vi "Set Result Collector.vi"(8 "error in (no error)":errorcluster, 10 "Report Generator":refnum<class "Result Collector.lvclass">, 11 "Icon Decorator In":refnum<class "Icon Decorator.lvclass">) -> (0 "error out":errorcluster, 3 "Icon Decorator Out":refnum<class "Icon Decorator.lvclass">)   [LabVIEW 2020, in "Icon Decorator.lvclass"]
uses:
  Icon Decorator.lvclass
  C:/Users/anton/Documents/GitHub/LUnit/source/Application Framework/Process Classes/Process/Process.lvclass
  Result Collector/Result Collector.lvclass
  Application Framework/Process Classes/Process/Process.lvclass/Process.ctl
  Application Framework/Process Classes/Process/Process.lvclass
  Result Classes/Method Result/Method Result.lvclass
  Result Classes/Test Case Result/Test Case Result.lvclass
  Result Classes/Test Suite Result/Test Suite Result.lvclass
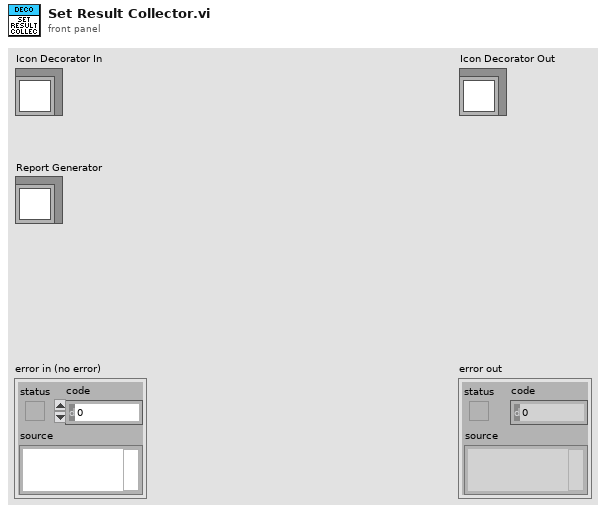
[diagram p1: front panel]
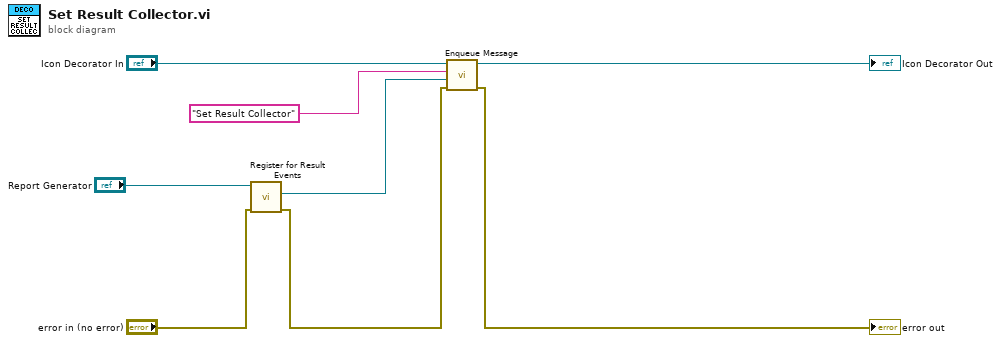
[diagram p0: block diagram]
diagram:
  n1 = call "Register for Result Events.vi"("error in (no error)"="error in (no error)", "Result Collector In"="Report Generator") -> ("error out"=w2:errorcluster, "Event Registration Refnum"=w3:refnum<event-registration>)  [unwired: 7 in, 1 out]
  n2 = call "Enqueue Message.vi"("error in (no error)"=w2, "Message Data"=w3, "Message"="Set Result Collector", "Process In"="Icon Decorator In") -> ("error out"=→"error out":errorcluster, "Process Out"=→"Icon Decorator Out":refnum<class "Icon Decorator.lvclass">)  [unwired: 6 in]
